vi "Read Txt File as Lines.vi"(8 "error in":errorcluster, 11 "file path (use dialog)":path) -> (0 "error out":errorcluster, 3 "Lines":string[](array[string]))   [LabVIEW 2014]
doc: "This Function is designed to read in a text file and retunr an array of string with each line of the text file. \n\nFor comments or questions about this code please look at the community example page below.\nhttp://decibel.ni.com/content/docs/DOC-10662"
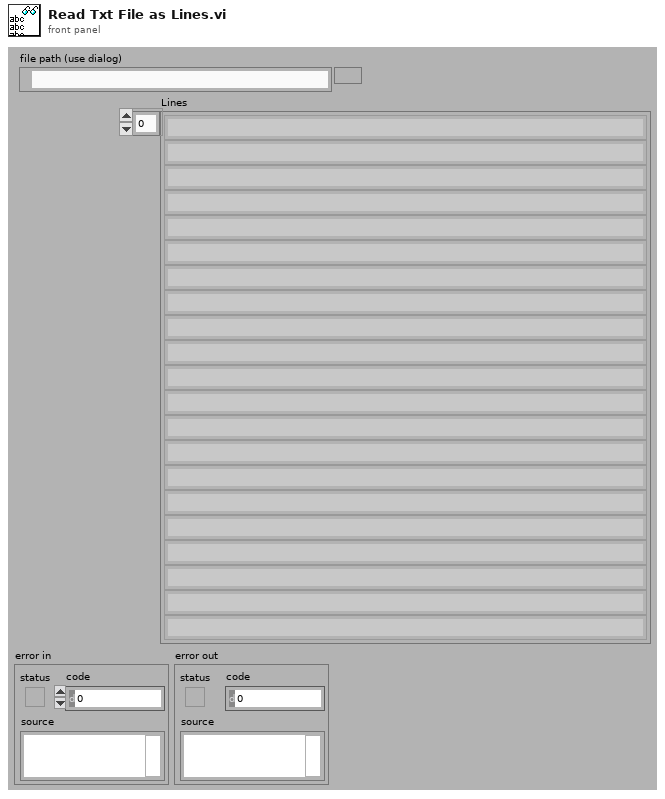
[diagram p1: front panel]
types:
  T1 = enum16{"open", "replace", "create", "open or create", "replace or create", "replace or create with confirmation"}
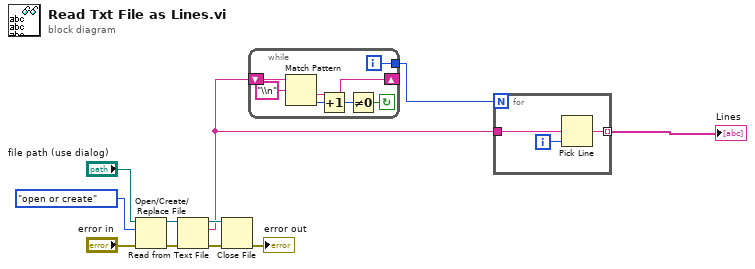
[diagram p0: block diagram]
diagram:
  n1 = Open/Create/Replace File(file path (use dialog)="file path (use dialog)", error in="error in", operation (0:open)=T1."open or create") -> (refnum out=w11:refnum<file>, error out=w10:errorcluster)  [unwired: 3 in, 1 out]
  n2 = Read from Text File(file (use dialog)=w11, error in=w10) -> (refnum out=w6:refnum<file>, text=w1:string, error out=w7:errorcluster)  [unwired: 2 in, 1 out]
  n3 = Close File(refnum=w6, error in=w7) -> (error out=→"error out":errorcluster)  [unwired: 1 out]
  n4 = while {
    tunnel: [w12] -> w2
    shift-left: w1 -> [w18]
    shift-right: [w16] -> _
    i -> [w12]
    stop <- w13 continue-if-true
    n5 = Match Pattern(string=w18, regular expression="\\n") -> (after substring=w16:string, offset past match=w15:i32)  [unwired: 1 in, 2 out]
    n6 = Increment(x=w15) -> (x+1=w14:i32)
    n7 = Not Equal To 0?(x=w14) -> (x != 0?=w13:bool)
  }
  n8 = for {
    N: w2 -> [_]
    tunnel: w1 -> [w20]
    tunnel: [w19] -> w5 mode=indexing
    i -> [w21]
    n9 = Pick Line(multi-line string=w20, line index=w21) -> (output string=w19:string)  [unwired: 1 in]
  }
  "Lines" <- w5
